vi "Test.vi"() -> ()   [LabVIEW 2018, in "Functions.lvlib" / "MultiBandState.lvclass"]
uses:
  MultiBandState.lvclass
  TypeDefs/clMultiBandConfig.ctl
  TypeDefs/MultiBandConfig.ctl
  X:/Projects/NistPluggableModules/dev/NistPluggableModules/FGen/MemberClasses/FunctionBaseClass/FunctionBase.lvclass
  <vilib>/Analysis/Matrix/Datatypes/RealMatrix.ctl
  MultiBandState.lvclass/MultiBandState.ctl
  FunctionBaseClass/FunctionBase.lvclass/FunctionBase.ctl
  Accessors/Read MultiBand.vi
  FunctionBaseClass/Accessors/Read Waveforms.vi
  Accessors/Write SampleRate.vi
  Accessors/Write MultiBand.vi
  Accessors/Write MultiBandConfig.vi
  <vilib>/Analysis/Matrix/NI_Matrix.lvlib
panel:
  in  "MultiBandConfig":T1
  out "Y":dbl[](graph)
  out "X(1)":dbl[](graph)
  # "Band"
  # "Band"
  # "Band"
  # "Band"
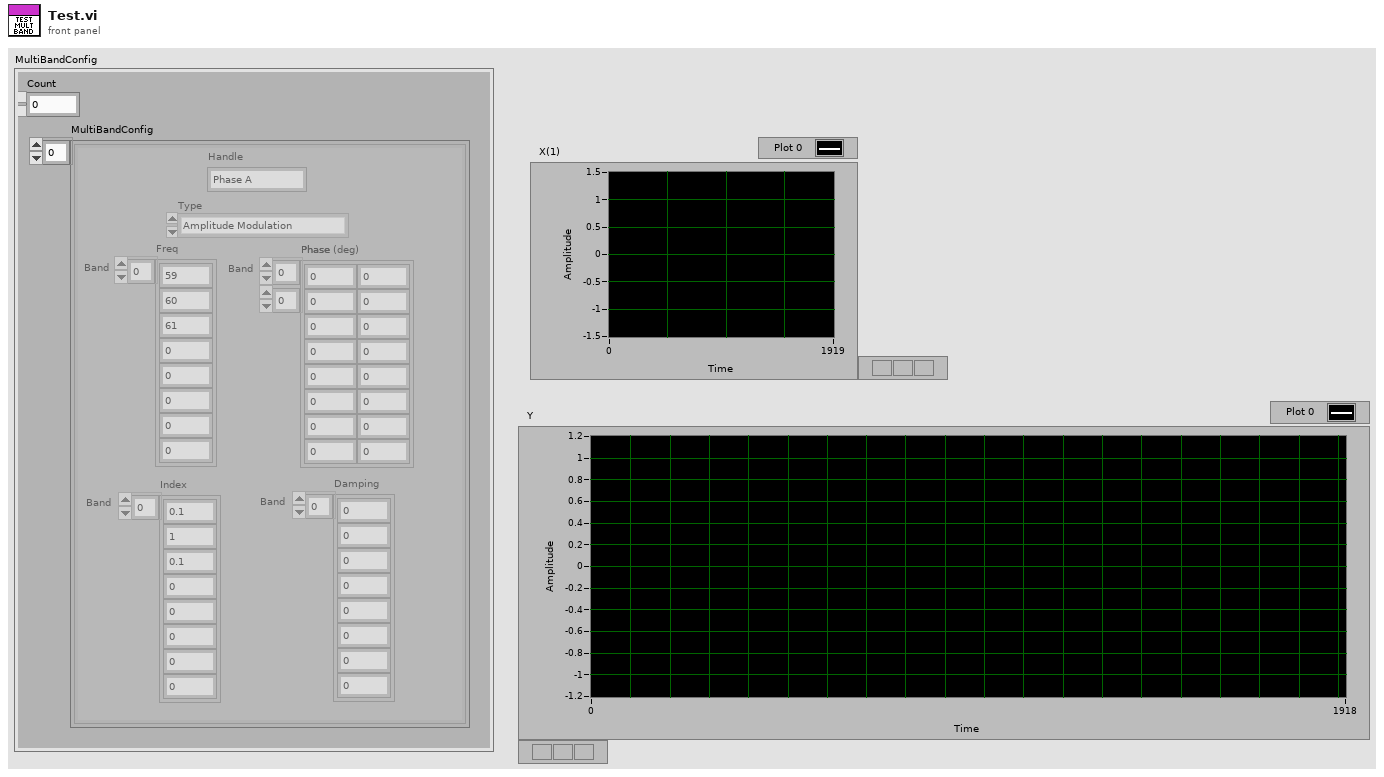
[diagram p1: front panel]
types:
  T1 = typedef "Functions.lvlib/MultiBandState.lvclass/clMultiBandConfig.ctl" = cluster{"Count":i32, "MultiBandConfig":T2[]}
  T2 = typedef "Functions.lvlib/MultiBandState.lvclass/MultiBandConfig.ctl" = cluster{"Handle":string, "Type":enum16{"Multiband", "Amplitude Modulation", "Phase Modulation", "Combined Modulation"}, "Freq":dbl[], "Index":dbl[], "Phase":dbl[][], "Damping":dbl[]}
  T3 = typedef "NI_Matrix.lvlib/RealMatrix.ctl" = dbl[][]
  T4 = cluster{"Handle":string, "Size":i32, "Gain":dbl, "Offset":dbl, "A":T3, "B":T3, "C":T3, "D":T3, "X":T3, "Waveform":waveform(dbl)}[]
  T5 = cluster{"Handle":string, "Size":i32, "Gain":dbl, "Offset":dbl, "A":T3, "B":T3, "C":T3, "D":T3, "X":T3, "Waveform":waveform(dbl)}
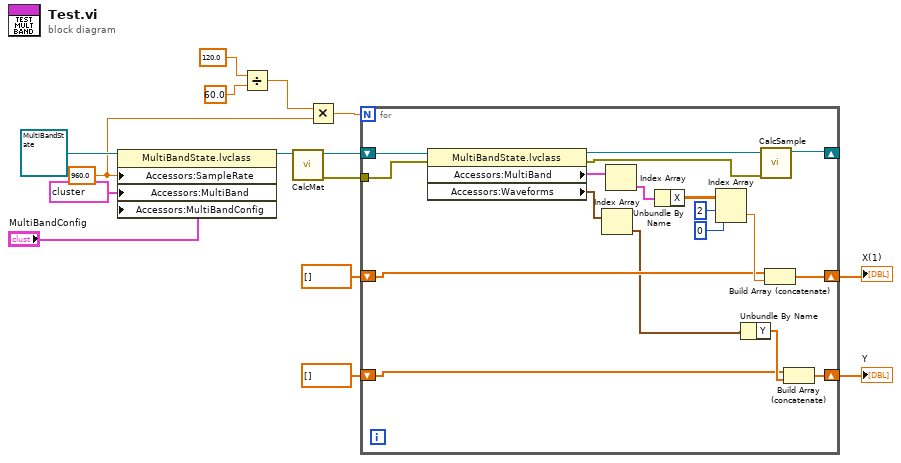
[diagram p0: block diagram]
diagram:
  w13 = 960.0 ("SampleRate")
  n1 = property class="MultiBandState.lvclass"(reference=refnum<class "MultiBandState.lvclass"> refnum ("MultiBandState in"), "Accessors:SampleRate"=w13, "Accessors:MultiBand"=T4 [{"Handle"="Foo", "Size"=0, "Gain"=0.0, "Offset"=0.0, "A"=[], "B"=[], "C"=[], "D"=[], "X"=[], "Waveform"={"t0"=timestamp(0 s since 1904-01-01), "dt"=1.0, "Y"=[]}}] ("MultiBand"), "Accessors:MultiBandConfig"="MultiBandConfig") -> (reference out=w14:refnum<class "MultiBandState.lvclass">)  [unwired: 1 in, 1 out]
  n2 = Divide(x=120.0, y=60.0) -> (x/y=w4:dbl)
  n3 = call "CalcMat.vi"("MultiBandState in"=w14) -> ("error out"=w10:errorcluster, "MultiBandState out"=w11:refnum<class "MultiBandState.lvclass">)  [unwired: 9 in]
  n4 = Multiply(x=w4, y=w13) -> (x*y=w12:dbl)
  n5 = for {
    N: w12 -> [_]
    tunnel: w10 -> [w19]
    shift-right: [w28] -> w9
    shift-left: dbl[] [] -> [w27]
    shift-right: [w21] -> _
    shift-left: w11 -> [w20]
    shift-right: [w24] -> w5
    shift-left: dbl[] [] -> [w23]
    n6 = property class="MultiBandState.lvclass"(reference=w20, error in=w19) -> (reference out=w22:refnum<class "MultiBandState.lvclass">, error out=w18:errorcluster, "Accessors:MultiBand"=w33:T4, "Accessors:Waveforms"=w17:waveform(dbl)[])
    n7 = Index Array(array=w17) -> (element=w16:waveform(dbl))  [unwired: 1 in]
    n8 = Index Array(array=w33) -> (element=w26:T5)  [unwired: 1 in]
    n9 = Unbundle By Name(w26) -> ("X"=w32:T3)
    n10 = Index Array(array=w32, index (row)=2, index (col)=0) -> (element=w29:dbl)
    n11 = Unbundle By Name(w16) -> ("Y"=w25:dbl[])
    n12 = call "CalcSample.vi"("error in (no error)"=w18, "MultiBandState in"=w22) -> ("MultiBandState out"=w21:refnum<class "MultiBandState.lvclass">)  [unwired: 8 in, 1 out]
    n13 = Build Array (concatenate)(w27, w29) -> (w28:dbl[])
    n14 = Build Array (concatenate)(w23, w25) -> (w24:dbl[])
  }
  "X(1)" <- w9
  "Y" <- w5
